vi "gugudan server.vi"() -> ()   [LabVIEW 2014]
panel:
  out "Client ip address":string="Client ip address"
  in  "사용설명서":bool
  out "로그인":bool
  in  "ID":string="ID"
  in  "PW":string="PW"
  in  "E-Mail":string="E-Mail  address"
  in  "명령전달":bool
  in  "address":string="ip address"
  out "명령코드":i16[](array[numeric])
  out "참 거짓":string="상태창입니다."
  out "문자열":string="명령창 입니다."
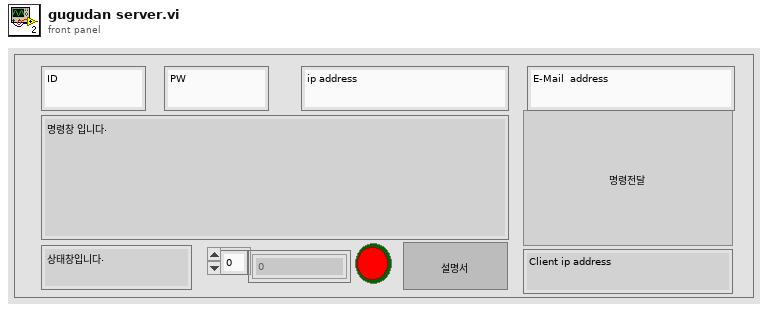
[diagram p1: front panel]
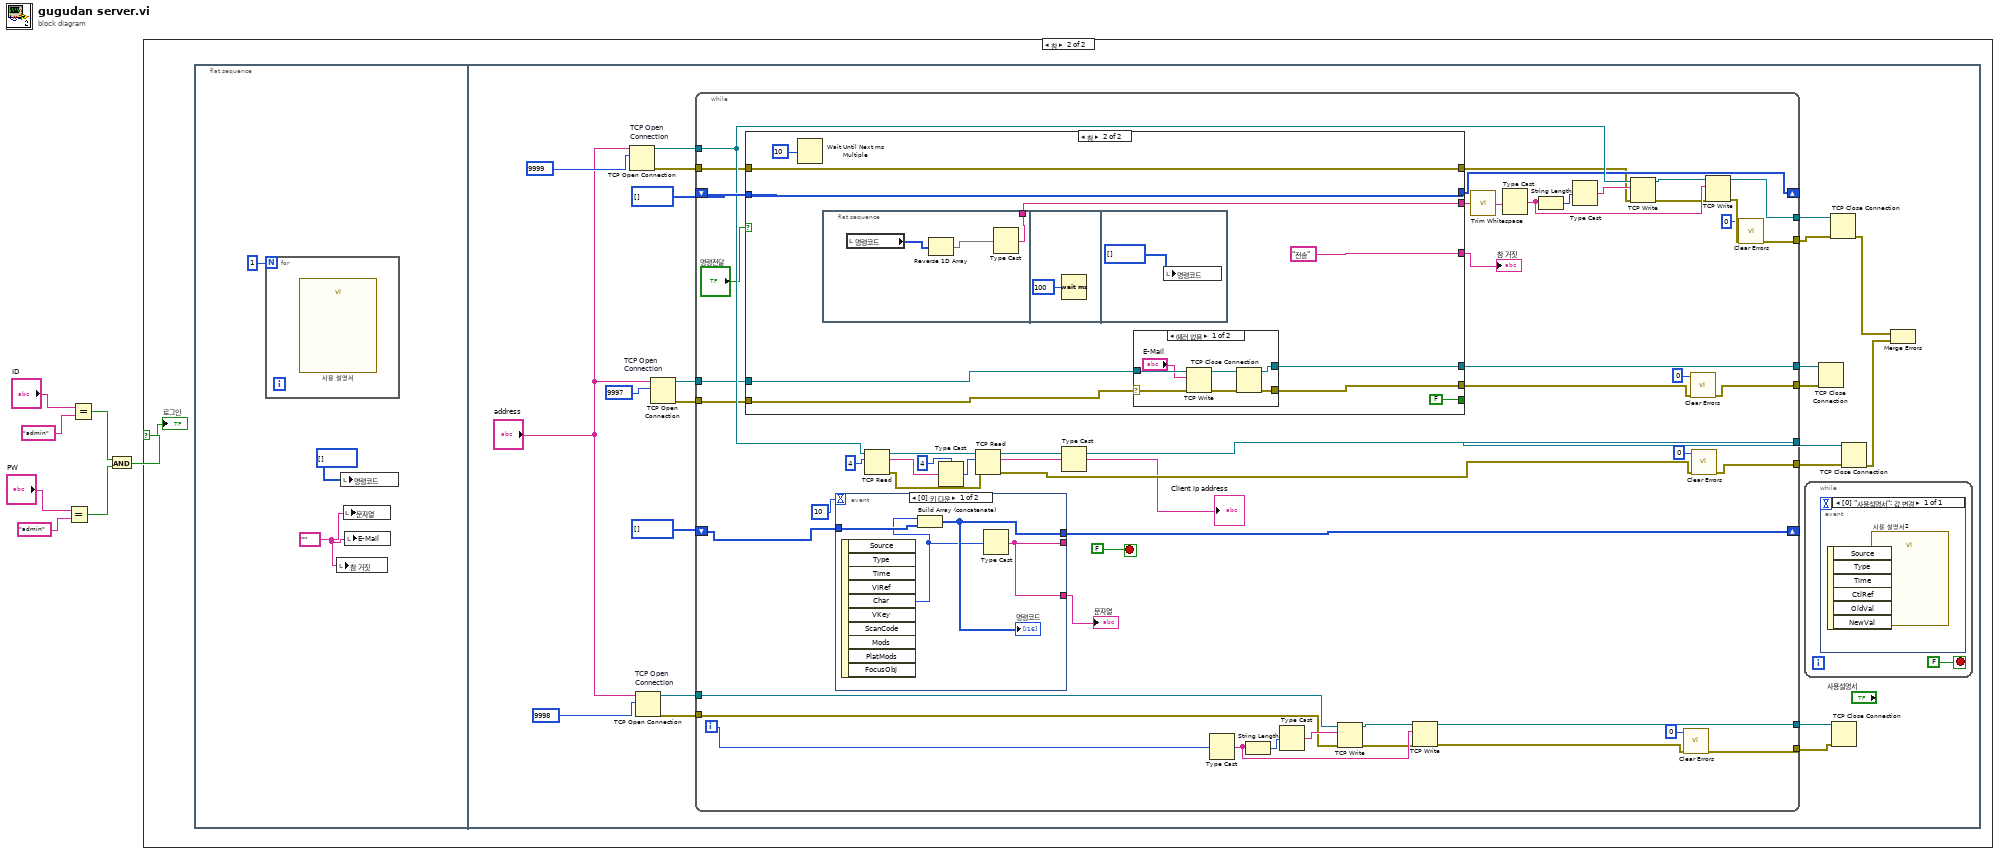
[diagram p0: block diagram]
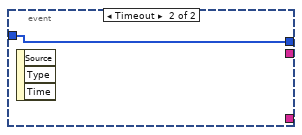
[diagram p3: hidden frame]
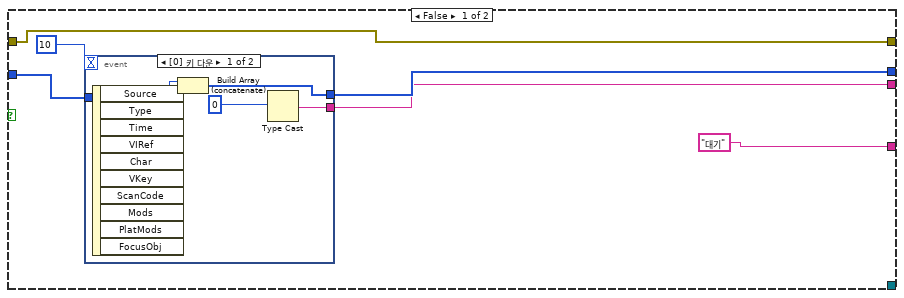
[diagram p4: hidden frame]
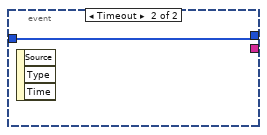
[diagram p5: hidden frame]
diagram:
  n1 = Equal?(x="PW", y="admin") -> (x = y?=w2:bool)
  n2 = Equal?(x="ID", y="admin") -> (x = y?=w3:bool)
  n3 = And(x=w3, y=w2) -> (x .and. y?=w1:bool)
  n4 = case shown="참" w1 {
    selector: w1 -> [_ w8]
    frame False {
    }
    frame True {
      n5 = flat-sequence {
        frame #0 {
          w10 = ""
          n6 = for {
            N: 1 -> [_]
            n7 = call "사용 설명서"() -> ()  [unwired: 10 in, 2 out]
          }
          n8 = local write "참 거짓"(w10) -> ()
          n9 = local write "명령코드"(i16[] []) -> ()
          n10 = local write "문자열"(w10) -> ()
          n11 = local write "E-Mail"(w10) -> ()
        }
        frame #1 {
          n12 = TCP Open Connection "TCP Open \nConnection"(address="address", remote port or service name=u16 9999) -> (connection ID=w33:refnum<k5>, error out=w27:errorcluster)  [unwired: 3 in]
          n13 = TCP Open Connection "TCP Open \nConnection"(address="address", remote port or service name=u16 9998) -> (connection ID=w22:refnum<k5>, error out=w19:errorcluster)  [unwired: 3 in]
          n14 = TCP Open Connection "TCP Open \nConnection"(address="address", remote port or service name=u16 9997 ("원격 포트 또는 서비스 이름")) -> (connection ID=w17:refnum<k5>, error out=w16:errorcluster)  [unwired: 3 in]
          n15 = while {
            tunnel: w33 -> [w80]
            tunnel: [w87] -> w31
            shift-right: [w69] -> _
            shift-left: i16[] [] -> [w86]
            tunnel: [w79] -> w30
            shift-right: [w70] -> _
            shift-left: i16[] [] -> [w71]
            tunnel: w27 -> [w68]
            tunnel: [w47] -> w13
            tunnel: [w44] -> w25
            tunnel: w22 -> [w55]
            tunnel: [w54] -> w21
            tunnel: [w42] -> w20
            tunnel: w19 -> [w53]
            tunnel: [w38] -> w18
            tunnel: w17 -> [w51]
            tunnel: w16 -> [w50]
            tunnel: [w49] -> w14
            i -> [w52]
            stop <- FALSE stop-if-true
            n16 = case shown="참" "명령전달" {
              tunnel: w86 -> [w98 w114]
              tunnel: [w97 w114] -> w69
              tunnel: [w95 w110] -> w63
              tunnel: w68 -> [w94 w112]
              tunnel: [w94 w112] -> w67
              tunnel: ["대기" "전송"] -> w62
              tunnel: [_ FALSE ("불리언")] -> _
              tunnel: [_ w108] -> w37
              tunnel: w51 -> [_ w107]
              tunnel: w50 -> [_ w106]
              tunnel: [_ w105] -> w49
              frame False {
                n17 = event shown="[0] 키 다운" {
                  selector: _ -> [_ _]
                  dyn-events: _ -> [_ _]
                  timeout: 10 -> [_ _]
                  tunnel: [w102 w104] -> w97
                  tunnel: w98 -> [w103 w104]
                  tunnel: [w100 _] -> w95
                  event Key Down {
                    n18 = event-data() -> ("Char"=w101:i16)  [unwired: 1 in, 9 out]
                    n19 = Build Array (concatenate)(w101, w103) -> (w102:i16[])
                    n20 = Type Cast(x=0) -> (*(type *) &x=w100:string)  [unwired: 1 in]
                  }
                  event Timeout {
                    n21 = event-data() -> ()  [unwired: 1 in, 3 out]
                  }
                }
              }
              frame True {
                n22 = Wait Until Next ms Multiple(millisecond multiple=u32 10) -> ()  [unwired: 1 out]
                n23 = flat-sequence {
                  tunnel: [w125] -> w110
                  frame #0 {
                    n24 = local read "명령코드"() -> (w126:i16[])
                    n25 = Reverse 1D Array(array=w126) -> (reversed array=w124:i16[])
                    n26 = Type Cast(x=w124) -> (*(type *) &x=w125:string)  [unwired: 1 in]
                  }
                  frame #1 {
                    n27 = Wait (ms)(milliseconds to wait=u32 100 ("대기 시간(ms)")) -> ()  [unwired: 1 out]
                  }
                  frame #2 {
                    n28 = local write "명령코드"(i16[] []) -> ()
                  }
                }
                n29 = case shown="에러 없음" w106 {
                  selector: w106 -> [w116 w123]
                  tunnel: [w120 w122] -> w105
                  tunnel: [w119 w123] -> w108
                  tunnel: w107 -> [w117 w122]
                  frame No Error {
                    n30 = TCP Write(connection ID=w117, data in="E-Mail", error in (no error)=w116) -> (connection ID out=w121:refnum<k5>, error out=w118:errorcluster)  [unwired: 2 out]
                    n31 = TCP Close Connection(connection ID=w121, error in (no error)=w118) -> (connection ID out=w120:refnum<k5>, error out=w119:errorcluster)  [unwired: 1 out]
                  }
                  frame Error {
                  }
                }
              }
            }
            "참 거짓" <- w62
            n32 = event shown="[0] 키 다운" {
              selector: _ -> [_ _]
              dyn-events: _ -> [_ _]
              timeout: 10 -> [_ _]
              tunnel: [w89 w92] -> w70
              tunnel: [w91 _] -> w72
              tunnel: [w91 _] -> _
              tunnel: w71 -> [w90 w92]
              event Key Down {
                n33 = event-data() -> ("Char"=w88:i16)  [unwired: 1 in, 9 out]
                n34 = Build Array (concatenate)(w88, w90) -> (w89:i16[])
                "명령코드" <- w89
                n35 = Type Cast(x=w88) -> (*(type *) &x=w91:string)  [unwired: 1 in]
              }
              event Timeout {
                n36 = event-data() -> ()  [unwired: 1 in, 3 out]
              }
            }
            "문자열" <- w72
            n37 = TCP Read(connection ID=w80, bytes to read=4) -> (connection ID out=w85:refnum<k5>, data out=w83:string, error out=w65:errorcluster)  [unwired: 3 in]
            n38 = Type Cast(type=4 ("bytes to read"), x=w83) -> (*(type *) &x=w82:i32)
            n39 = TCP Read(connection ID=w85, bytes to read=w82, error in (no error)=w65) -> (connection ID out=w79:refnum<k5>, data out=w81:string, error out=w43:errorcluster)  [unwired: 2 in]
            n40 = Type Cast(x=w81) -> (*(type *) &x=→"Client ip address":string)  [unwired: 1 in]
            n41 = Type Cast(x=w52) -> (*(type *) &x=w57:string)  [unwired: 1 in]
            n42 = String Length(string=w57) -> (length=w58:i32)
            n43 = Type Cast(x=w58) -> (*(type *) &x=w59:string)  [unwired: 1 in]
            n44 = TCP Write(connection ID=w55, data in=w59, error in (no error)=w53) -> (connection ID out=w60:refnum<k5>, error out=w56:errorcluster)  [unwired: 1 in, 1 out]
            n45 = TCP Write(connection ID=w60, data in=w57, error in (no error)=w56) -> (connection ID out=w54:refnum<k5>, error out=w41:errorcluster)  [unwired: 1 in, 1 out]
            n46 = call <vilib>:"Trim Whitespace.vi"("string"=w63) -> ("trimmed string"=w64:string)  [unwired: 1 in]
            n47 = Type Cast(x=w64) -> (*(type *) &x=w74:string)  [unwired: 1 in]
            n48 = String Length(string=w74) -> (length=w75:i32)
            n49 = Type Cast(x=w75) -> (*(type *) &x=w76:string)  [unwired: 1 in]
            n50 = TCP Write(connection ID=w80, data in=w76, error in (no error)=w67) -> (connection ID out=w77:refnum<k5>, error out=w66:errorcluster)  [unwired: 1 in, 1 out]
            n51 = call <vilib>:"Clear Errors.vi"("error in (no error)"=w41, "specific error code to clear (0: all)"=0) -> ("error out"=w42:errorcluster)  [unwired: 4 in, 1 out]
            n52 = call <vilib>:"Clear Errors.vi"("error in (no error)"=w37, "specific error code to clear (0: all)"=0) -> ("error out"=w38:errorcluster)  [unwired: 4 in, 1 out]
            n53 = call <vilib>:"Clear Errors.vi"("error in (no error)"=w43, "specific error code to clear (0: all)"=0) -> ("error out"=w44:errorcluster)  [unwired: 4 in, 1 out]
            n54 = TCP Write(connection ID=w77, data in=w74, error in (no error)=w66) -> (connection ID out=w87:refnum<k5>, error out=w46:errorcluster)  [unwired: 1 in, 1 out]
            n55 = call <vilib>:"Clear Errors.vi"("error in (no error)"=w46, "specific error code to clear (0: all)"=0) -> ("error out"=w47:errorcluster)  [unwired: 4 in, 1 out]
          }
          n56 = while {
            stop <- FALSE stop-if-true
            n57 = event shown="[0] \"사용설명서\": 값 변경" {
              selector: _ -> [_]
              dyn-events: _ -> [_]
              timeout: _ -> [_]
              event "사용설명서": Value Change {
                n58 = event-data() -> ()  [unwired: 1 in, 6 out]
                n59 = call "사용 설명서2"() -> ()  [unwired: 10 in, 2 out]
              }
            }
          }
          n60 = TCP Close Connection(connection ID=w14, error in (no error)=w18) -> ()  [unwired: 3 out]
          n61 = TCP Close Connection(connection ID=w31, error in (no error)=w13) -> (error out=w26:errorcluster)  [unwired: 1 in, 1 out]
          n62 = TCP Close Connection(connection ID=w21, error in (no error)=w20) -> ()  [unwired: 1 in, 2 out]
          n63 = TCP Close Connection(connection ID=w30, error in (no error)=w25) -> (error out=w24:errorcluster)  [unwired: 1 in, 1 out]
          n64 = Merge Errors(w26, w24) -> ()  [unwired: 1 out]
        }
      }
      "로그인" <- w8
    }
  }
